vi "Configure Logging.vi"(11 "File Path/File Name":string="/U/metrics.csv") -> (3 "refnum out":refnum<file>)   [LabVIEW 2015]
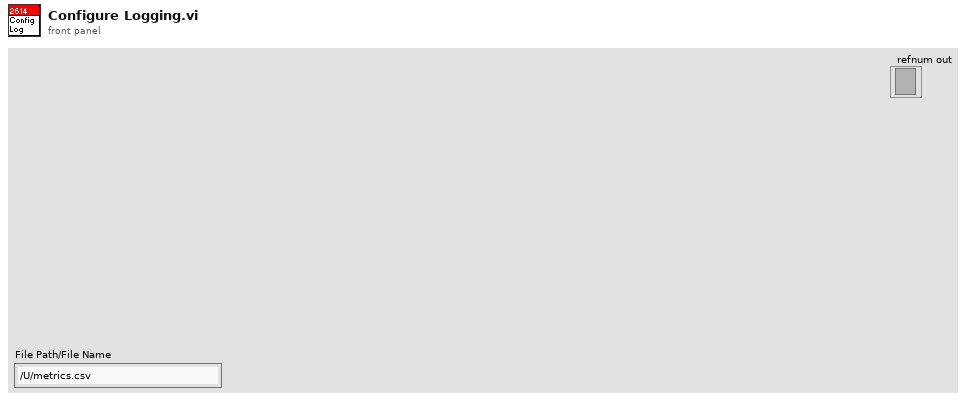
[diagram p1: front panel]
types:
  T1 = enum16{"open", "replace", "create", "open or create", "replace or create", "replace or create with confirmation"}
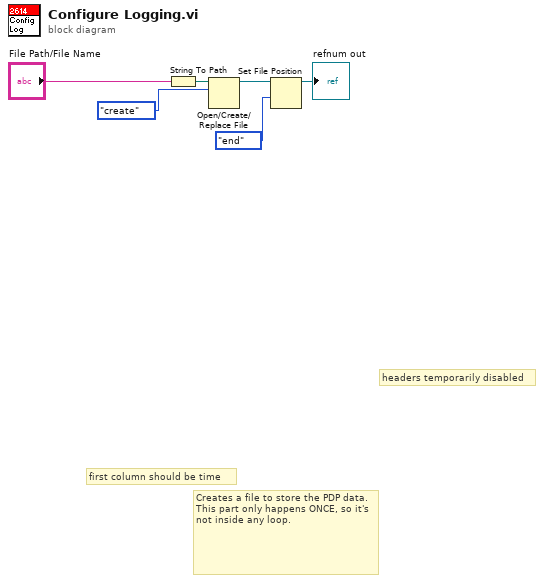
[diagram p0: block diagram]
diagram:
  # "headers temporarily disabled"
  # "first column should be time"
  # "Creates a file to store the PDP data. This part only happens ONCE, so it's not inside any loop."
  n1 = String To Path(string="File Path/File Name") -> (path=w5:path)
  n2 = Open/Create/Replace File(file path (use dialog)=w5, operation (0:open)=T1."create") -> (refnum out=w4:refnum<file>)  [unwired: 4 in, 2 out]
  n3 = Set File Position(refnum=w4, from (0:start)=enum16{"start", "end", "current"}."end") -> (refnum out=→"refnum out":refnum<file>)  [unwired: 2 in, 1 out]
